vi "Check for Valid Device.vi"(8 "error in (no error)":errorcluster, 11 "device in":refnum<class "NI_Robotics_Starter Kit Base Device.lvclass">) -> (0 "error out":errorcluster, 2 "valid?":bool, 3 "device out":refnum<class "NI_Robotics_Starter Kit Base Device.lvclass">)   [LabVIEW 2017, in "NI_Robotics_Starter Kit Base Device.lvclass"]
uses:
  <vilib>/robotics/Starter Kit/Base Device/NI_Robotics_Starter Kit Base Device.lvclass
  <vilib>/robotics/Starter Kit/Base Device/NI_Robotics_Starter Kit Base Device.lvclass/NI_Robotics_Starter Kit Base Device.ctl
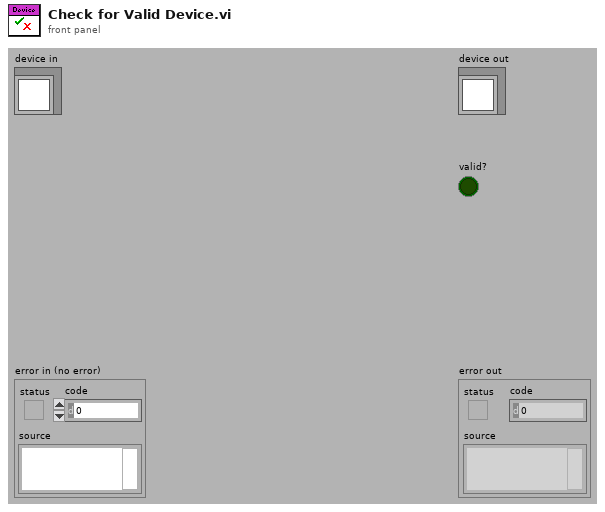
[diagram p1: front panel]
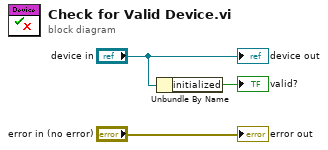
[diagram p0: block diagram]
diagram:
  n1 = Unbundle By Name("device in") -> ("initialized"=→"valid?":bool)
  "error out" <- "error in (no error)"
  "device out" <- "device in"
